vi "ReadSweep.vi"(8 "error in (no error)":errorcluster, 10 "channel":string, 11 "map":T1) -> (0 "error out":errorcluster, 1 "sweep":cluster{"frequency":dbl, "amplitude":dbl}[](array[cluster]), 2 "found":bool, 3 "map out":T1, 4 "unit":string, 5 "valid":bool)   [LabVIEW 2017, in "EmsaAcquisition.lvlib"]
uses:
  <vilib>/addons/InsightCM/Devices/Shared/Emsa/EmsaAcquisition/EmsaAcquisition.lvlib
  <vilib>/addons/PointValueMap/controls/PointMap.ctl
  <vilib>/addons/PointValueMap/subVIs/Point_Read_string.vi
  <vilib>/addons/PointValueMap/PointValueMap.lvlib
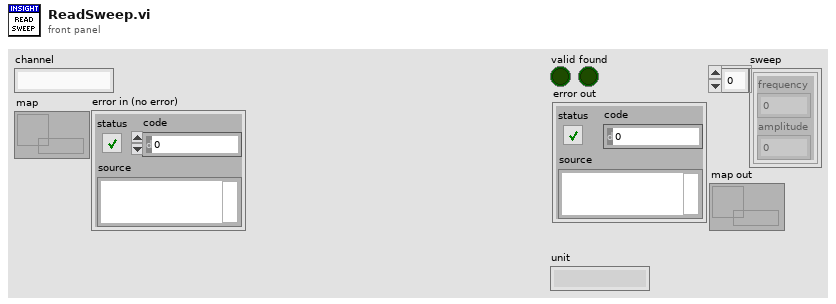
[diagram p1: front panel]
types:
  T1 = typedef "PointValueMap.lvlib/PointMap.ctl" = refnum<data-value>
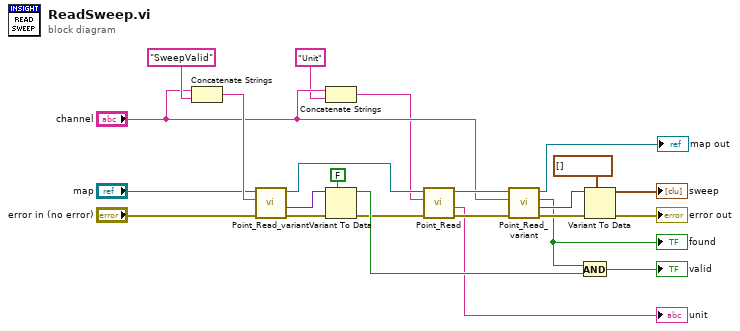
[diagram p0: block diagram]
diagram:
  n1 = Concatenate Strings("channel", "SweepValid" ("Tag")) -> (w20:string)
  n2 = call <vilib>:"Point_Read_variant.vi"("Error In"="error in (no error)", "Tag"=w20, "Map"="map") -> ("Error Out"=w21:errorcluster, "Value"=w23:variant, "Map Out"=w8:T1)  [unwired: 3 in, 3 out]
  n3 = Concatenate Strings("channel", "Unit" ("Tag")) -> (w1:string)
  n4 = Variant To Data(error in=w21, type=FALSE, Variant=w23) -> (data=w13:bool, error out=w6:errorcluster)
  n5 = call-poly <vilib>:"Point_Read.vi"("Error In"=w6, "Tag"=w1, "Map"=w8) -> ("Error Out"=w5:errorcluster, "Value"=→"unit":string, "Map Out"=w7:T1)  [unwired: 3 in, 3 out]
  n6 = call <vilib>:"Point_Read_variant.vi"("Error In"=w5, "Tag"="channel", "Map"=w7) -> ("Error Out"=w15:errorcluster, "Value"=w17:variant, "Found?"=w14:bool, "Map Out"=→"map out":T1)  [unwired: 3 in, 2 out]
  "found" <- w14
  n7 = And(x=w14, y=w13) -> (x .and. y?=→"valid":bool)
  n8 = Variant To Data(error in=w15, type=cluster{"frequency":dbl, "amplitude":dbl}[] [] ("sweep"), Variant=w17) -> (data=→"sweep":cluster{"frequency":dbl, "amplitude":dbl}[], error out=→"error out":errorcluster)
